vi "运维调试_总磷总氮.vi"() -> ()   [LabVIEW 2016, in "斯坦道总氮.lvlib"]
uses:
  <vilib>/Utility/miscctls.llb/LVPointTypeDef.ctl
  <vilib>/Plasmionique/MB Master/MB_Master/MB_Master.lvclass
  <vilib>/Utility/config.llb/NI_LVConfig.lvlib
  <vilib>/ptbypt/NI_PtbyPt.lvlib
panel:
  in  "关闭心跳包":bool
  out "权限等级":enum16{"一级权限", "二级权限", "三级权限", "超级权限"}(ring)
  out "试剂余量显示":sgl[][](graph)
  in  "仪器校准":bool
  in  "参数查询":bool
  out "简易步骤名称":string
  in  "温度曲线":bool
  in  "试剂余量":bool
  in  "灯值调整":bool
  in  "启动参数设置":bool
  out "固件版本号":string
  in  "定时设置":cluster{"启动":bool, "控制命令":T1, "测量参数":T2}(xcontrol)
  out "模块版本号":string
  out "注射器温度":sgl
  out "消解温度":sgl
  out "ADC":sgl
  out "F3":sgl format="%#.6f"
  out "F2":sgl format="%#.6f"
  out "F1":sgl format="%#.6f"
  out "F0":sgl format="%#.6f"
  out "运行状态":T3 {"数据时间:" format="%<%y/%m/%d %H:%M:%S>T"; "仪器时间:" format="%<%y/%m/%d %H:%M:%S>T"}
  in  "单选按钮":T4(radio)=enum."总氮"
  out "布尔":bool
  in  "流程固件":bool
  out "字符串 2":string
  in  "数组":string[](array[string])
  in  "返回":bool
  in  "参数设置":bool
  out "集成报警信息":string
  in  "停止":bool
  in  "手动启动":bool
  in  "调试":bool
  out "多列列表框":i32(listbox)
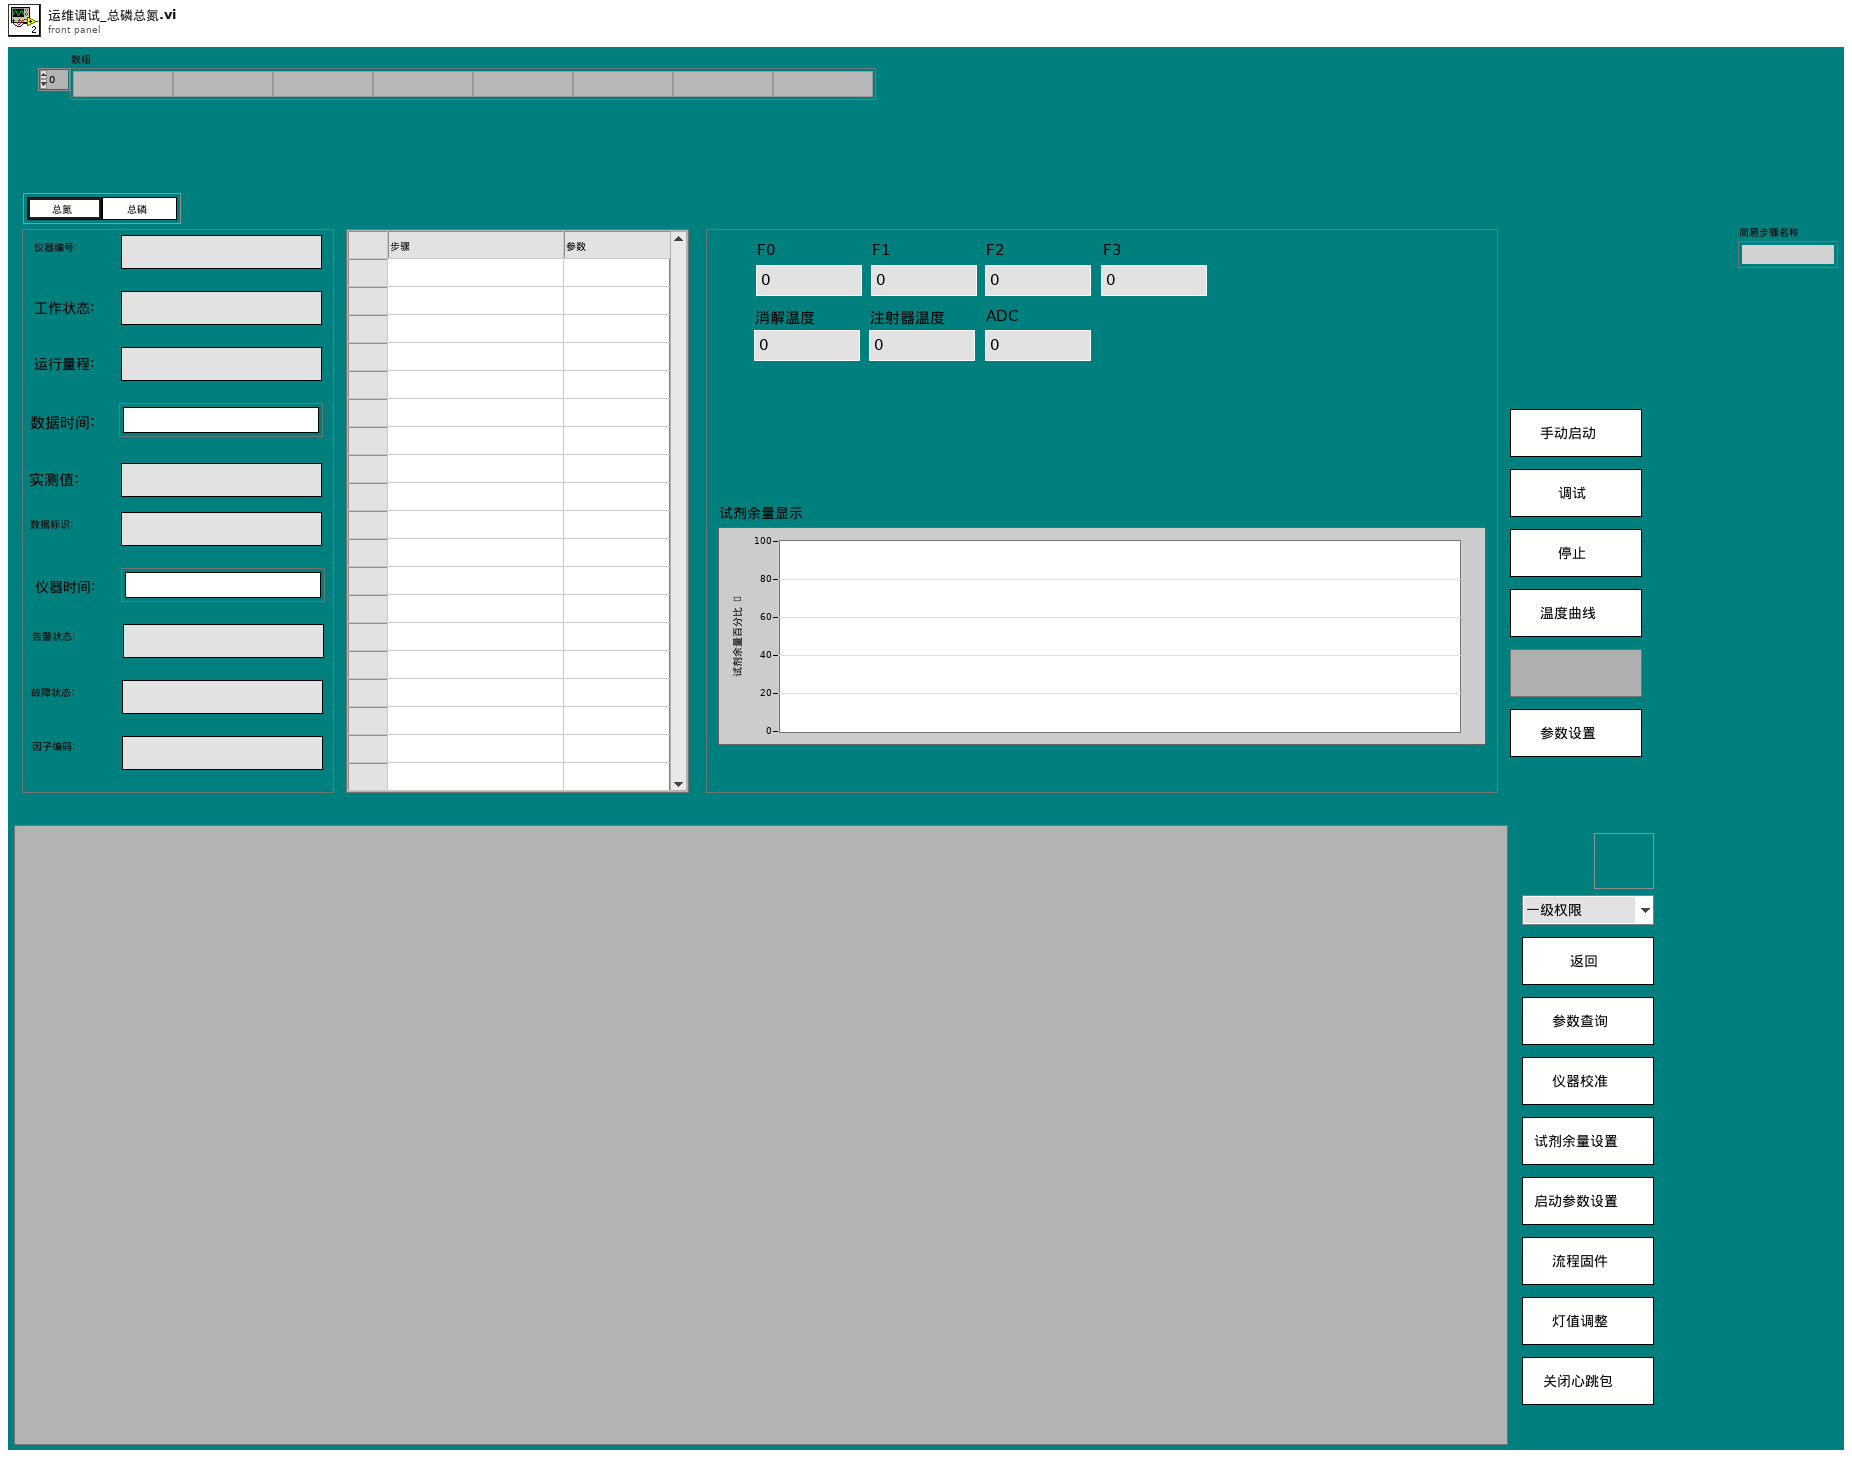
[diagram p1: front panel]
types:
  T1 = typedef "定时设置.xctl/国标控制命令.ctl" = enum16{"启动测量", "标样核查", "零点核查", "跨度核查", "空白测试", "平行样测试", "加标回收", "空白校准", "标样校准", "初始化（清洗）", "停止测试", "仪器重启", "校时", "模式设置", "测量间隔设置"}
  T2 = typedef "定时设置.xctl/测量参数.ctl" = u16
  T3 = cluster{"仪器编号:":string, "工作状态:":string, "运行量程: ":string, "数据时间:":timestamp, "实测值:":string, "数据标识: ":string, "仪器时间:":timestamp, "告警状态: ":string, "故障状态:  ":string, "因子编码:":string}
  T4 = enum32{"COD", "氨氮", "总氮", "总磷", "磷酸盐", "硝氮", "亚硝氮", "硅酸盐", "硫化物"}
  T5 = cluster{"时间源选择":enum16{"系统时间源", "仪器时间源"}, "外部时间源":timestamp}
  T6 = cluster{"系统时间":timestamp, "工作状态":u16, "测量模式":enum16{"待机", "连续模式", "周期模式", "定点模式", "受控模式", "手动模式"}, "告警代码":u16, "故障代码":u16, "日志代码":u16, "软件版本":u16, "F0":sgl, "F1":sgl, "F2":sgl, "F3":sgl, "T":sgl, "H":sgl, "id":u16, "flowid":u16, "量程":u16, "总磷控温温度1":sgl, "营养盐控温温度2":sgl, "ADC":sgl}
  T7 = enum32{"Bad", "Idle", "Run top level", "Running"}
  T8 = typedef "LVPointTypeDef.ctl" = cluster{"Horizontal":i16, "Vertical":i16}
  T9 = cluster{"因子编码":u32, "单位":u16, "标样参考值":sgl, "水样数据时间":timestamp, "水样实测值":sgl, "水样数据标识":string, "标样数据时间":timestamp, "标样实测值":sgl, "标样数据标识":string, "空白数据时间":timestamp, "空白实测值":sgl, "空白数据标识":string, "零点核查数据时间":timestamp, "零点核查实测值":sgl, "零点核查数据标识":string, "跨度核查数据时间":timestamp, "跨度核查实测值":sgl, "跨度核查数据标识":string, "加标回收数据时间":timestamp, "加标回收实测值":sgl, "加标回收数据标识":string, "平行样数据时间":timestamp, "平行样实测值":sgl, "平行样数据标识":string, "F0":sgl, "F1":sgl, "F2":sgl, "F3":sgl, "F4":sgl, "F5":sgl, "F6":sgl, "F7":sgl, "温度":sgl, "湿度":sgl, "X值":sgl, "fidrange":u16}[]
  T10 = cluster{"因子编码":u32, "单位":u16, "标样参考值":sgl, "水样数据时间":timestamp, "水样实测值":sgl, "水样数据标识":string, "标样数据时间":timestamp, "标样实测值":sgl, "标样数据标识":string, "空白数据时间":timestamp, "空白实测值":sgl, "空白数据标识":string, "零点核查数据时间":timestamp, "零点核查实测值":sgl, "零点核查数据标识":string, "跨度核查数据时间":timestamp, "跨度核查实测值":sgl, "跨度核查数据标识":string, "加标回收数据时间":timestamp, "加标回收实测值":sgl, "加标回收数据标识":string, "平行样数据时间":timestamp, "平行样实测值":sgl, "平行样数据标识":string, "F0":sgl, "F1":sgl, "F2":sgl, "F3":sgl, "F4":sgl, "F5":sgl, "F6":sgl, "F7":sgl, "温度":sgl, "湿度":sgl, "X值":sgl, "fidrange":u16}
  T11 = cluster{"时间标识":timestamp, "设备":string, "日志信息":string, "备注":string}
  T12 = cluster{"参数":string, "报警内容":string, "报警分析":string}
  T13 = cluster{"Major":u16, "Minor":u16, "Fix":u16, "Build":u16}
  T14 = typedef "NI_LVConfig.lvlib/Config Data RefNum.ctl" = refnum<k1>
  T15 = cluster{"时间标识":timestamp, "设备":string, "日志信息":string, "流程参数":string}
  T16 = typedef "LVRowAndColumnUnsignedTypeDef.ctl" = cluster{"Row":u32, "Column":u32}
  T17 = enum16{"空闲", "水样测试", "标样核查", "零点核查", "跨度核查", "空白测试", "平行样测试", "加标回收", "空白校准", "标样校准", "初始化（清洗）"}
  T18 = cluster{"站号":u16, "量程切换":enum32{"H", "L", "AUTO"}, "控制命令":enum16{"启动测量", "标样核查", "零点核查", "跨度核查", "空白测试", "平行样测试", "加标回收", "空白校准", "标样校准", "初始化（清洗）", "停止测试", "仪器重启", "校时", "模式设置", "测量间隔设置"}, "模式设置":enum16{"待机", "连续模式", "周期模式", "定点模式", "受控模式", "手动模式"}, "测量间隔":u16}
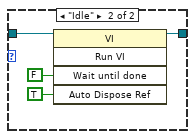
[diagram p4: hidden frame]
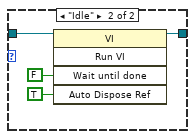
[diagram p5: hidden frame]
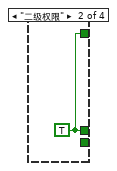
[diagram p13: hidden frame]
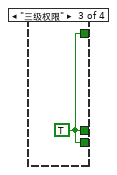
[diagram p14: hidden frame]
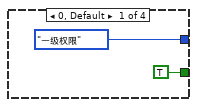
[diagram p15: hidden frame]
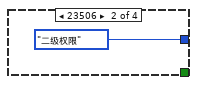
[diagram p16: hidden frame]
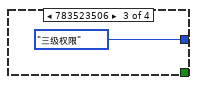
[diagram p17: hidden frame]
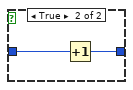
[diagram p19: hidden frame]
diagram:
  n1 = while {
    stop <- FALSE stop-if-true
    n2 = vi-ref "测量流程.vi"() -> (w49:refnum<vi>)
    n3 = global read "VAR总磷总氮全局变量.vi" "状态告警区"() -> (w46:T6)
    n4 = Wait (ms)(milliseconds to wait=u32 500 ("等待时间（毫秒）")) -> ()  [unwired: 1 out]
    n5 = Unbundle By Name("定时设置") -> ("启动"=w43:bool, "控制命令"=w42:T1)
    n6 = property class="VI"(reference=w49) -> ("Exec.State"=w48:T7, "Name"=w47:string)  [unwired: 1 in, 2 out]
    n7 = Unbundle By Name(w46) -> ("工作状态"=w45:u16, "系统时间"=w40:timestamp)
    n8 = case shown="真" w43 {
      tunnel: w47 -> [_ w56]
      tunnel: w42 -> [_ w55]
      tunnel: w48 -> [_ w54]
      frame False {
      }
      frame True {
        n9 = case shown="\"Idle\"" w54 {
          tunnel: w56 -> [_ w60]
          tunnel: w55 -> [_ w57]
          frame "Bad", Default {
          }
          frame "Idle" {
            n10 = Open VI Reference(type specifier VI Refnum (for type only)=refnum<vi> refnum, vi path=w60, options=128 ("选项")) -> (vi reference=w61:refnum<vi>, error out=w62:errorcluster)  [unwired: 3 in]
            n11 = call-by-ref "开始异步调用"(reference=w61, error in=w62, "控制命令"=w57) -> (reference out=w63:refnum<vi>, error out=w64:errorcluster)  [unwired: 11 in]
            n12 = Close Reference(reference=w63, error in (no error)=w64) -> ()  [unwired: 1 out]
          }
        }
      }
    }
    n13 = case shown="1, 默认" w45 {
      tunnel: [FALSE TRUE] -> w38
      frame 0 {
      }
      frame 1, Default {
      }
    }
    n14 = Bundle By Name(cluster=T5 {"时间源选择"=enum."仪器时间源", "外部时间源"=timestamp(0 s since 1904-01-01)} ("时间源"), "外部时间源"=w40) -> (w39:T5)
    n15 = property on="定时设置" class="定时设置 (严格)"("仪器状态"=w38, "时间源"=w39) -> ()  [unwired: 2 in, 2 out]
  }
  n16 = control-ref of="本VI"() -> (w20:refnum<vi>)
  n17 = call "配置文件路径.vi"() -> ("appended path"=w31:path)  [unwired: 11 in]
  n18 = call "时间延迟"() -> ("error out"=w37:errorcluster)  [unwired: 11 in]
  n19 = flat-sequence {
    frame #0 {
      n20 = property on="窗格" class="Pane"("Origin"=T8 {"Horizontal"=0, "Vertical"=0} ("原点")) -> ()  [unwired: 2 in, 2 out]
    }
  }
  n21 = while {
    shift-right: [w68] -> _
    shift-left: _ -> [w67]
    stop <- FALSE stop-if-true
    n22 = global write "VAR总磷总氮全局变量.vi" "最近一次工作状态"(w67) -> ()
    n23 = global read "VAR总磷总氮全局变量.vi" "状态告警区"() -> (w90:T6)
    n24 = global read "VAR总磷总氮全局变量.vi" "通讯状态"() -> (w101:bool)
    n25 = Wait (ms)(milliseconds to wait=u32 1000 ("等待时间（毫秒）")) -> ()  [unwired: 1 out]
    n26 = case shown="\"COD\", 默认" "单选按钮" {
      tunnel: [22 3 2 1 4 5 6 7 8] -> w69
      frame "COD", Default {
      }
      frame "氨氮" {
      }
      frame "总氮" {
      }
      frame "总磷" {
      }
      frame "磷酸盐" {
      }
      frame "硝氮" {
      }
      frame "亚硝氮" {
      }
      frame "硅酸盐" {
      }
      frame "硫化物" {
      }
    }
    n27 = Unbundle By Name(w90) -> ("id"=w89:u16, "工作状态"=w84:u16)
    n28 = case shown="真" w101 {
      tunnel: ["通讯异常" ("集成报警信息") w195] -> w100
      frame False {
      }
      frame True {
        n29 = global read "VAR总磷总氮全局变量.vi" "状态告警区"() -> (w201:T6)
        n30 = Unbundle By Name(w201) -> ("工作状态"=w200:u16)
        n31 = feedback #1(0) -> (w198:i32)
        n32 = case shown="默认" w200 {
          tunnel: w198 -> [_ w203]
          tunnel: [_ w202] -> w196
          frame 0 {
          }
          frame Default {
            n33 = Increment(x=w203) -> (x+1=w202:i32)
          }
        }
        n34 = feedback-in #1(w196) -> ()
        n35 = global read "VAR总磷总氮全局变量.vi" "测量状态"() -> (w194:string)
        n36 = Format Into String(format string="工作计时: %d 秒" ("格式字符串"), initial string=w194, w196) -> (resulting string=w195:string)  [unwired: 1 in, 1 out]
      }
    }
    "集成报警信息" <- w100
    n37 = global read "VAR总磷总氮全局变量.vi" "测量数据区数组"() -> (w73:T9)
    n38 = case shown="1, 默认" w84 {
      tunnel: w89 -> [_ w146]
      frame 0 {
      }
      frame 1, Default {
        n39 = case shown="8" w146 {
          frame 0, Default {
          }
          frame 1 {
            n40 = local write "单选按钮"(T4."总磷" ("单选按钮")) -> ()
          }
          frame 2 {
            n41 = local write "单选按钮"(T4."总氮" ("单选按钮")) -> ()
          }
          frame 22 {
            n42 = local write "单选按钮"(T4."COD" ("单选按钮")) -> ()
          }
          frame 3 {
            n43 = local write "单选按钮"(T4."氨氮" ("单选按钮")) -> ()
          }
          frame 4 {
            n44 = local write "单选按钮"(T4."磷酸盐" ("单选按钮")) -> ()
          }
          frame 5 {
            n45 = local write "单选按钮"(T4."硝氮" ("单选按钮")) -> ()
          }
          frame 6 {
            n46 = local write "单选按钮"(T4."亚硝氮" ("单选按钮")) -> ()
          }
          frame 7 {
            n47 = local write "单选按钮"(T4."硅酸盐" ("单选按钮")) -> ()
          }
          frame 8 {
            n48 = local write "单选按钮"(T4."硫化物" ("单选按钮")) -> ()
          }
        }
      }
    }
    n49 = call "id参数转换.vi"("id"=w69) -> ("数组资源索引"=w70:i32)  [unwired: 9 in, 1 out]
    n50 = global read "VAR总磷总氮全局变量.vi" "状态告警区"() -> (w99:T6)
    n51 = Index Array(array=w73, index=w70) -> (element=w72:T10)
    n52 = Unbundle By Name(w99) -> ("系统时间"=w95:timestamp, "工作状态"=w94:u16, "告警代码"=w88:u16, "故障代码"=w86:u16, "量程"=w93:u16)
    n53 = case shown="5, 8" w67 {
      tunnel: [w115 w121 w125 w129 w133 w137 w141 w145] -> w83
      tunnel: [w113 w120 w124 w128 w131 w136 w140 w144] -> w78
      tunnel: [w116 w119 w123 w127 w130 w135 w139 w143] -> w76
      tunnel: w72 -> [_ w118 w122 w126 w132 w134 w138 w142]
      frame 0, Default {
        n54 = local read "运行状态"() -> (w117:T3)
        n55 = Unbundle By Name(w117) -> ("数据时间:"=w115:timestamp, "实测值:"=w114:string, "数据标识:"=w116:string)
        n56 = Fract/Exp String To Number(string=w114) -> (number=w113:dbl)  [unwired: 3 in, 1 out]
      }
      frame 1 {
        n57 = Unbundle By Name(w118) -> ("水样数据时间"=w121:timestamp, "水样实测值"=w120:sgl, "水样数据标识"=w119:string)
      }
      frame 2, 9 {
        n58 = Unbundle By Name(w122) -> ("标样数据时间"=w125:timestamp, "标样实测值"=w124:sgl, "标样数据标识"=w123:string)
      }
      frame 3 {
        n59 = Unbundle By Name(w126) -> ("零点核查数据时间"=w129:timestamp, "零点核查实测值"=w128:sgl, "零点核查数据标识"=w127:string)
      }
      frame 4 {
        n60 = Unbundle By Name(w132) -> ("跨度核查数据时间"=w133:timestamp, "跨度核查实测值"=w131:sgl, "跨度核查数据标识"=w130:string)
      }
      frame 7 {
        n61 = Unbundle By Name(w134) -> ("加标回收数据时间"=w137:timestamp, "加标回收实测值"=w136:sgl, "加标回收数据标识"=w135:string)
      }
      frame 5, 8 {
        n62 = Unbundle By Name(w138) -> ("空白数据时间"=w141:timestamp, "空白实测值"=w140:sgl, "空白数据标识"=w139:string)
      }
      frame 6 {
        n63 = Unbundle By Name(w142) -> ("平行样数据时间"=w145:timestamp, "平行样实测值"=w144:sgl, "平行样数据标识"=w143:string)
      }
    }
    n64 = Unbundle By Name(w72) -> ("因子编码"=w74:u32)
    n65 = case shown="255" w94 {
      selector: w94 -> [w160 _ w166 w168 w170 w172 w174 w176 w178 w180 w182 w184 w186 w188]
      tunnel: [w161 "空闲" ("工作状态") "水样测量" ("工作状态") "标样核查" ("工作状态") "零点核查" ("工作状态") "跨度核查" ("工作状态") "空白测试" ("工作状态") "平行样测试" ("工作状态") "加标回收" ("工作状态") "空白校准" ("工作状态") "标样校准" ("工作状态") "初始化" ("工作状态") "单步调试" ("工作状态") w190] -> w66
      tunnel: [w159 w164 w166 w168 w170 w172 w174 w176 w178 w180 w182 w184 w186 w188] -> w68
      tunnel: w67 -> [w159 w164 _ _ _ _ _ _ _ _ _ _ _ _]
      frame Default {
        n66 = Format Into String(format string="%d" ("格式字符串"), initial string="未知" ("工作状态"), w160) -> (resulting string=w161:string)  [unwired: 1 in, 1 out]
      }
      frame 0 {
      }
      frame 1 {
      }
      frame 2 {
      }
      frame 3 {
      }
      frame 4 {
      }
      frame 5 {
      }
      frame 6 {
      }
      frame 7 {
      }
      frame 8 {
      }
      frame 9 {
      }
      frame 10 {
      }
      frame 254 {
      }
      frame 255 {
        n67 = local read "简易步骤名称"() -> (w191:string)
        n68 = Format Into String(format string="-%d (%s)" ("格式字符串"), initial string="简易流程" ("工作状态"), w188, w191) -> (resulting string=w190:string)  [unwired: 1 in, 1 out]
      }
    }
    n69 = case shown="1" w93 {
      tunnel: ["" ("字符串") "低量程 " ("字符串") "高量程 " ("字符串")] -> w92
      frame Default {
      }
      frame 0 {
      }
      frame 1 {
      }
    }
    n70 = Number To Fractional String(number=w78, precision (6)=i16 4 ("精度(6)")) -> (F-format string=w80:string)  [unwired: 2 in]
    n71 = Concatenate Strings(w80, " " ("字符串"), "mg/L" ("字符串")) -> (w77:string)
    n72 = global read "VAR总磷总氮全局变量.vi" "序列号"() -> (w96:string)
    n73 = Format Into String(format string="w%05d" ("格式字符串"), w74) -> (resulting string=w91:string)  [unwired: 2 in, 1 out]
    n74 = call "告警码字段定义.vi"("告警代码"=w88) -> ("字符串"=w87:string)  [unwired: 8 in, 2 out]
    n75 = call "故障码字段定义.vi"("故障代码"=w86) -> ("字符串"=w85:string)  [unwired: 10 in]
    n76 = global write "VAR总磷总氮全局变量.vi" "工作状态:"(w66) -> ()
    n77 = Bundle By Name(cluster=T3 {"仪器编号:"="", "工作状态:"="", "运行量程: "="", "数据时间:"=timestamp(0 s since 1904-01-01), "实测值:"="", "数据标识: "="", "仪器时间:"=timestamp(0 s since 1904-01-01), "告警状态: "="", "故障状态:  "="", "因子编码:"=""} ("运行状态"), "仪器编号:"=w96, "仪器时间:"=w95, "工作状态:"=w66, "告警状态:"=w87, "故障状态:"=w85, "运行量程:"=w92, "数据时间:"=w83, "实测值:"=w77, "数据标识:"=w76, "因子编码:"=w91) -> (→"运行状态":T3)
  }
  n78 = call "Create balloon 队列.vi"() -> ("队列输出"=w34:refnum<queue>)  [unwired: 11 in]
  n79 = while {
    shift-right: [w207] -> _
    shift-left: _ -> [w206]
    stop <- FALSE stop-if-true
    n80 = global read "VAR总磷总氮全局变量.vi" "状态告警区"() -> (w209:T6)
    n81 = Wait (ms)(milliseconds to wait=u32 1000 ("等待时间（毫秒）")) -> ()  [unwired: 1 out]
    n82 = Unbundle By Name(w209) -> ("工作状态"=w208:u16, "总磷控温温度1"=w205:sgl, "营养盐控温温度2"=w204:sgl)
    n83 = case shown="默认" w208 {
      tunnel: [TRUE _] -> w207
      tunnel: w206 -> [w218 _]
      tunnel: w205 -> [w216 _]
      tunnel: w204 -> [w214 _]
      frame Default {
        n84 = case shown="真" w218 {
          tunnel: [_ w221] -> w217
          tunnel: [_ w220] -> w215
          frame False {
          }
          frame True {
            n85 = global read "VAR总磷总氮全局变量.vi" "波形图-消解温度"() -> (w221:dbl[])
            n86 = global read "VAR总磷总氮全局变量.vi" "波形图-注射器温度"() -> (w220:dbl[])
          }
        }
        n87 = Insert Into Array(array=w217, new element=w216) -> (w213:dbl[])  [unwired: 1 in]
        n88 = Insert Into Array(array=w215, new element=w214) -> (w212:dbl[])  [unwired: 1 in]
        n89 = global write "VAR总磷总氮全局变量.vi" "波形图-消解温度"(w213) -> ()
        n90 = global write "VAR总磷总氮全局变量.vi" "波形图-注射器温度"(w212) -> ()
      }
      frame 0, 254, 255 {
      }
    }
  }
  n91 = while {
    stop <- FALSE stop-if-true
    n92 = control-ref of="试剂余量显示"() -> (w223:refnum<vi>)
    n93 = Wait (ms)(milliseconds to wait=u32 10000 ("等待时间（毫秒）")) -> ()  [unwired: 1 out]
    n94 = call "试剂余量展示.vi"("波形图 2"=w223) -> ("波形图"=→"试剂余量显示":sgl[][])  [unwired: 10 in]
  }
  n95 = call "试剂余量后台任务.vi"() -> ()  [unwired: 12 in]
  n96 = while {
    shift-right: [w238] -> _
    shift-left: u32 0 ("y") -> [w240]
    stop <- FALSE stop-if-true
    # "密码权限"
    n97 = local read "布尔"() -> (w241:bool)
    n98 = global read "VAR总磷总氮全局变量.vi" "权限密码"() -> (w233:u32)
    n99 = global read "VAR总磷总氮全局变量.vi" "权限等级"() -> (w230:enum16{"一级权限", "二级权限", "三级权限", "超级权限"})
    n100 = global read "VAR总磷总氮全局变量.vi" "权限等级"() -> (→"权限等级":enum16{"一级权限", "二级权限", "三级权限", "超级权限"})
    n101 = Wait (ms)(milliseconds to wait=u32 1000 ("等待时间（毫秒）")) -> ()  [unwired: 1 out]
    n102 = case shown="假" w241 {
      tunnel: w240 -> [_ w254]
      tunnel: [_ w253] -> w238
      frame False {
      }
      frame True {
        n103 = Increment(x=w254) -> (x+1=w253:u32)
      }
    }
    n104 = case shown="783523103" w233 {
      tunnel: [enum16{"一级权限", "二级权限", "三级权限", "超级权限"}."一级权限" ("权限等级") enum16{"一级权限", "二级权限", "三级权限", "超级权限"}."二级权限" ("权限等级") enum16{"一级权限", "二级权限", "三级权限", "超级权限"}."三级权限" ("权限等级") enum16{"一级权限", "二级权限", "三级权限", "超级权限"}."超级权限" ("权限等级")] -> w234
      tunnel: [TRUE _ _ _] -> w232
      frame 0, Default {
      }
      frame 23506 {
      }
      frame 783523506 {
      }
      frame 783523103 {
      }
    }
    n105 = case shown="\"超级权限\"" w230 {
      tunnel: [_ w243 w244 w246] -> w227
      tunnel: [_ _ w244 w246] -> w229
      tunnel: [_ w243 w244 w246] -> w228
      tunnel: [_ _ _ TRUE] -> w226
      frame "一级权限", Default {
      }
      frame "二级权限" {
        w243 = TRUE
      }
      frame "三级权限" {
        w244 = TRUE
      }
      frame "超级权限" {
        w246 = TRUE
      }
    }
    n106 = Greater Or Equal?(x=w238, y=u32 3600) -> (x >= y?=w236:bool)
    n107 = property on="关闭心跳包" class="Bool (严格)"("Visible"=w226) -> ()  [unwired: 2 in, 2 out]
    n108 = case shown="真" w236 {
      frame False {
      }
      frame True {
        n109 = global write "VAR总磷总氮全局变量.vi" "权限密码"(u32 0 ("权限密码")) -> ()
      }
    }
    n110 = property on="流程固件" class="Bool"("Visible"=w228) -> ()  [unwired: 2 in, 2 out]
    n111 = property on="试剂余量" class="Bool"("Visible"=w227) -> ()  [unwired: 2 in, 2 out]
    n112 = property on="灯值调整" class="Bool"("Visible"=w227) -> ()  [unwired: 2 in, 2 out]
    n113 = property on="启动参数设置" class="Bool"("Visible"=w229) -> ()  [unwired: 2 in, 2 out]
    n114 = global write "VAR总磷总氮全局变量.vi" "权限等级"(w234) -> ()
    n115 = Not(x=w232) -> (.not. x?=→"布尔":bool)
  }
  n116 = while {
    tunnel: w34 -> [w261]
    shift-right: [w257] -> _
    shift-left: _ -> [w258]
    stop <- FALSE stop-if-true
    n117 = global read "VAR总磷总氮全局变量.vi" "状态告警区"() -> (w255:T6)
    n118 = Wait (ms)(milliseconds to wait=u32 100) -> ()  [unwired: 1 out]
    n119 = Unbundle By Name(w255) -> ("工作状态"=w256:u16, "id"=w263:u16, "日志代码"=w262:u16, "故障代码"=w260:u16, "告警代码"=w259:u16)
    n120 = case shown="1, 默认" w256 {
      tunnel: w263 -> [_ w278]
      tunnel: w262 -> [_ w277]
      tunnel: w261 -> [_ w274]
      tunnel: w260 -> [_ w273]
      tunnel: w259 -> [_ w272]
      tunnel: w258 -> [w266 w271]
      tunnel: [w266 w270] -> w257
      frame 0 {
      }
      frame 1, Default {
        n121 = call "id参数转换.vi"("id"=w278) -> ("table输出"=w275:string)  [unwired: 9 in, 1 out]
        n122 = Add(x=w273, y=w272) -> (x+y=w270:u16)
        n123 = Not Equal?(x=w270, y=w271) -> (x != y?=w268:bool)
        n124 = Not Equal To 0?(x=w270) -> (x != 0?=w269:bool)
        n125 = call "故障告警分析.vi"("告警代码"=w272, "故障代码"=w273, "运行步序"=w277, "参数"=w275) -> ("报警内容"=w276:T12)  [unwired: 6 in, 1 out]
        n126 = And(x=w269, y=w268) -> (x .and. y?=w267:bool)
        n127 = case shown="真" w267 {
          tunnel: w276 -> [_ w287]
          tunnel: w274 -> [_ w286]
          frame False {
          }
          frame True {
            n128 = Unbundle By Name(w287) -> ("参数"=w282:string, "报警内容"=w281:string, "报警分析"=w280:string)
            n129 = Get Date/Time In Seconds() -> (seconds since 1Jan1904=w285:timestamp)
            n130 = Bundle("报警内容"=w281, "报警分析"=w280) -> (w279:cluster{"报警内容":string, "报警分析":string})  [unwired: 1 in]
            n131 = Bundle By Name(cluster=T11 {"时间标识"=timestamp(0 s since 1904-01-01), "设备"="", "日志信息"="", "备注"=""} ("data in"), "时间标识"=w285, "设备"=w282, "日志信息"=w281, "备注"=w280) -> (w284:T11)
            n132 = call "balloon入队列.vi"("报警内容"=w279, "队列"=w286) -> ()  [unwired: 9 in, 1 out]
            n133 = call "总磷总氮报警信息.vi"("data in"=w284) -> ()  [unwired: 10 in, 1 out]
          }
        }
      }
    }
  }
  n134 = Read from Text File(file (use dialog)=w31) -> (text=w32:string)  [unwired: 3 in, 3 out]
  n135 = flat-sequence {
    tunnel: [w289] -> w26
    tunnel: [w288] -> w24
    tunnel: w26 -> [w300]
    tunnel: [w300] -> w25
    tunnel: w24 -> [_]
    tunnel: w25 -> [w330]
    tunnel: [w330] -> w27
    tunnel: w27 -> [w333]
    tunnel: [w403] -> w28
    tunnel: [errorcluster {"status"=FALSE, "code"=0, "source"=""} ("错误输入（无错误）")] -> w3
    tunnel: [errorcluster {"status"=FALSE, "code"=0, "source"=""} ("错误输入（无错误）")] -> w2
    frame #0 {
      n136 = call "配置读取.vi"() -> ("error out"=w288:errorcluster)  [unwired: 11 in]
      n137 = control-ref of="本VI"() -> (w299:refnum<vi>)
      n138 = property class="VI"(reference=w299) -> ("Library.Version"=w298:T13)  [unwired: 1 in, 2 out]
      n139 = Unbundle By Name(w298) -> ("Major"=w296:u16, "Minor"=w295:u16, "Fix"=w294:u16, "Build"=w293:u16)
      n140 = control-ref of="本VI"() -> (w290:refnum<vi>)
      n141 = property class="VI"(reference=w290) -> ("Library"=w291:refnum<vi>)  [unwired: 1 in, 2 out]
      n142 = Format Into String(format string="模块版本号：%d.%d.%d.%d" ("格式字符串"), w296, w295, w294, w293) -> (resulting string=→"模块版本号":string)  [unwired: 2 in, 1 out]
      n143 = property class="Library"(reference=w291) -> ("LocalName"=w289:string)  [unwired: 1 in, 2 out]
      n144 = property on="定时设置" class="定时设置 (严格)"("引用参数"=w289) -> ()  [unwired: 2 in, 2 out]
    }
    frame #1 {
      n145 = global read "总磷总氮断电保存全局变量.vi" "IP"() -> (w304:string)
      n146 = global read "总磷总氮断电保存全局变量.vi" "VISA Resource"() -> (w301:refnum<visa-resource-name>)
      n147 = Empty String/Path?(string/path=w304) -> (empty?=w303:bool)
      n148 = case shown="真" w303 {
        tunnel: w300 -> [_ w315]
        frame False {
        }
        frame True {
          n149 = case shown="\"斯坦道CODcr.lvlib\"" w315 {
            tunnel: [w316 "192.168.1.203" ("IP") "192.168.1.202" ("IP") "192.168.1.202" ("IP") "192.168.1.203" ("IP") "192.168.1.204" ("IP") "192.168.1.205" ("IP")] -> w314
            frame Default {
              n150 = global read "总磷总氮断电保存全局变量.vi" "IP"() -> (w316:string)
            }
            frame "斯坦道总磷总氮.lvlib" {
            }
            frame "斯坦道氨氮.lvlib" {
            }
            frame "斯坦道氨氮总磷.lvlib" {
            }
            frame "斯坦道总磷.lvlib" {
            }
            frame "斯坦道总氮.lvlib" {
            }
            frame "斯坦道CODcr.lvlib" {
            }
          }
          n151 = global write "总磷总氮断电保存全局变量.vi" "IP"(w314) -> ()
        }
      }
      n152 = Empty String/Path?(string/path=w301) -> (empty?=w302:bool)
      n153 = case shown="真" w302 {
        tunnel: w300 -> [_ w306]
        frame False {
        }
        frame True {
          n154 = case shown="\"斯坦道总氮.lvlib\"" w306 {
            tunnel: [w307 "COM5" ("IP") "COM7" ("IP") "COM7" ("IP") "COM5" ("IP") "COM10" ("IP") "COM9" ("IP")] -> w305
            frame Default {
              n155 = global read "总磷总氮断电保存全局变量.vi" "VISA Resource"() -> (w307:refnum<visa-resource-name>)
            }
            frame "斯坦道总磷总氮.lvlib" {
            }
            frame "斯坦道氨氮.lvlib" {
            }
            frame "斯坦道氨氮总磷.lvlib" {
            }
            frame "斯坦道总磷.lvlib" {
            }
            frame "斯坦道总氮.lvlib" {
            }
            frame "斯坦道CODcr.lvlib" {
            }
          }
          n156 = global write "总磷总氮断电保存全局变量.vi" "VISA Resource"(w305) -> ()
        }
      }
    }
    frame #2 {
      n157 = global read "总磷总氮断电保存全局变量.vi" "MB通信方式选择"() -> (w326:enum16{"串口", "TCP"})
      n158 = global read "总磷总氮断电保存全局变量.vi" "VISA Resource"() -> (w325:refnum<visa-resource-name>)
      n159 = global read "总磷总氮断电保存全局变量.vi" "PORT"() -> (w328:string)
      n160 = Decimal String To Number(string=w328) -> (number=w327:i32)  [unwired: 2 in, 1 out]
      n161 = global read "总磷总氮断电保存全局变量.vi" "IP"() -> (w329:string)
      n162 = call "获取启动参数.vi"("MB通信方式选择"=w326, "Port (502)"=w327, "IP Address"=w329, "VISA Resource"=w325) -> ("error out"=w324:errorcluster, "数组"=w323:cluster{"String":string, "Value":u16}[])  [unwired: 6 in]
      n163 = case shown="无错误" w324 {
        tunnel: w323 -> [w331 _]
        frame No Error {
          n164 = flat-sequence {
            tunnel: w331 -> [w332]
            frame #0 {
              n165 = global write "总磷总氮断电保存全局变量.vi" "启动队列名称"(w332) -> ()
            }
            frame #1 {
              n166 = call "配置写入.vi"() -> ()  [unwired: 11 in, 1 out]
            }
          }
        }
        frame Error {
        }
      }
    }
    frame #3 {
      n167 = global read "总磷总氮断电保存全局变量.vi" "启动队列名称"() -> (w335:cluster{"String":string, "Value":u16}[])
      n168 = Empty Array?(array=w335) -> (empty?=w334:bool)
      n169 = case shown="真" w334 {
        tunnel: w333 -> [_ w336]
        frame False {
        }
        frame True {
          n170 = case shown="\"斯坦道总氮.lvlib\"" w336 {
            frame Default {
            }
            frame "斯坦道总磷总氮.lvlib" {
              n171 = global write "总磷总氮断电保存全局变量.vi" "启动队列名称"(cluster{"String":string, "Value":u16}[] [{"String"="总氮", "Value"=2}, {"String"="总磷", "Value"=1}] ("启动队列名称")) -> ()
            }
            frame "斯坦道氨氮.lvlib" {
              n172 = global write "总磷总氮断电保存全局变量.vi" "启动队列名称"(cluster{"String":string, "Value":u16}[] [{"String"="氨氮", "Value"=3}] ("启动队列名称")) -> ()
            }
            frame "斯坦道氨氮总磷.lvlib" {
              n173 = global write "总磷总氮断电保存全局变量.vi" "启动队列名称"(cluster{"String":string, "Value":u16}[] [{"String"="氨氮", "Value"=3}, {"String"="总磷", "Value"=1}] ("启动队列名称")) -> ()
            }
            frame "斯坦道总磷.lvlib" {
              n174 = global write "总磷总氮断电保存全局变量.vi" "启动队列名称"(cluster{"String":string, "Value":u16}[] [{"String"="总磷", "Value"=1}] ("启动队列名称")) -> ()
            }
            frame "斯坦道总氮.lvlib" {
              n175 = global write "总磷总氮断电保存全局变量.vi" "启动队列名称"(cluster{"String":string, "Value":u16}[] [{"String"="总氮", "Value"=2}] ("启动队列名称")) -> ()
            }
            frame "斯坦道CODcr.lvlib" {
              n176 = global write "总磷总氮断电保存全局变量.vi" "启动队列名称"(cluster{"String":string, "Value":u16}[] [{"String"="CODcr", "Value"=22}] ("启动队列名称")) -> ()
            }
          }
        }
      }
    }
    frame #4 {
      # "初始化"
      n177 = global read "总磷总氮断电保存全局变量.vi" "简易流程路径"() -> (w344:path)
      n178 = global read "总磷总氮断电保存全局变量.vi" "流程路径"() -> (w347:path)
      n179 = global read "总磷总氮断电保存全局变量.vi" "启动队列名称"() -> (w357:cluster{"String":string, "Value":u16}[])
      n180 = global read "总磷总氮断电保存全局变量.vi" "启动队列名称"() -> (w355:cluster{"String":string, "Value":u16}[])
      n181 = call <vilib>:"Check if File or Folder Exists.vi"("path"=w347) -> ("file or folder exists?"=w352:bool)  [unwired: 8 in, 2 out]
      n182 = call <vilib>:"Check if File or Folder Exists.vi"("path"=w344) -> ("file or folder exists?"=w351:bool)  [unwired: 8 in, 2 out]
      n183 = for {
        tunnel: w357 -> [w374] mode=indexing
        tunnel: [w373] -> w356 mode=indexing
        n184 = Unbundle By Name(w374) -> ("String"=w373:string)
      }
      n185 = Not(x=w351) -> (.not. x?=w346:bool)
      n186 = Not(x=w352) -> (.not. x?=w350:bool)
      n187 = Empty String/Path?(string/path=w344) -> (empty?=w343:bool)
      n188 = for {
        tunnel: w355 -> [w372] mode=indexing
        shift-right: [w371] -> w354
        shift-left: "" -> [w369]
        n189 = Unbundle By Name(w372) -> ("String"=w370:string)
        n190 = Concatenate Strings(w369, w370) -> (w371:string)
      }
      n191 = Empty String/Path?(string/path=w347) -> (empty?=w348:bool)
      n192 = Or(x=w343, y=w346) -> (x .or. y?=w345:bool)
      n193 = Or(x=w348, y=w350) -> (x .or. y?=w349:bool)
      n194 = property on="单选按钮" class="RadioBtnsControl (严格)"() -> ("Controls[]"=w358:refnum<vi>[])  [unwired: 2 in, 2 out]
      n195 = for {
        tunnel: w358 -> [w382] mode=indexing
        tunnel: w356 -> [w381]
        n196 = property class="Ctl"(reference=w382) -> (reference out=w380:refnum<vi>, "Label.Text"=w376:string)  [unwired: 1 in, 1 out]
        n197 = case shown="\"COD\"" w376 {
          selector: w376 -> [w383 _]
          tunnel: [w383 "CODcr"] -> w375
          frame Default {
          }
          frame "COD" {
          }
        }
        n198 = Search 1D Array(1D array=w381, element=w375) -> (index of element=w379:i32)  [unwired: 1 in]
        n199 = Not Equal?(x=w379, y=-1) -> (x != y?=w377:bool)
        n200 = property class="Ctl"(reference=w380, "Visible"=w377) -> ()  [unwired: 1 in, 2 out]
      }
      n201 = case shown="真" w345 {
        frame False {
        }
        frame True {
          n202 = global read "总磷总氮断电保存全局变量.vi" "启动队列名称"() -> (w360:cluster{"String":string, "Value":u16}[])
          n203 = for {
            tunnel: w360 -> [w363] mode=indexing
            tunnel: [w362] -> w359 mode=indexing
            n204 = Unbundle By Name(w363) -> ("String"=w362:string)
          }
          n205 = call "获取默认流程路径.vi"("参数"=w359) -> ("路径"=w361:path)  [unwired: 10 in]
          n206 = global write "总磷总氮断电保存全局变量.vi" "简易流程路径"(w361) -> ()
        }
      }
      n207 = case shown="真" w349 {
        frame False {
        }
        frame True {
          n208 = global read "总磷总氮断电保存全局变量.vi" "启动队列名称"() -> (w365:cluster{"String":string, "Value":u16}[])
          n209 = for {
            tunnel: w365 -> [w368] mode=indexing
            tunnel: [w367] -> w364 mode=indexing
            n210 = Unbundle By Name(w368) -> ("String"=w367:string)
          }
          n211 = call "获取默认流程路径.vi"("参数"=w364) -> ("路径"=w366:path)  [unwired: 10 in]
          n212 = global write "总磷总氮断电保存全局变量.vi" "流程路径"(w366) -> ()
        }
      }
      n213 = global write "VAR总磷总氮全局变量.vi" "模块名称"(w354) -> ()
    }
    frame #5 {
      n214 = vi-ref "总磷总氮通讯.vi"() -> (w385:refnum<vi>)
      n215 = vi-ref "总磷总氮测量数据储存.vi"() -> (w393:refnum<vi>)
      n216 = property class="VI"(reference=w385) -> ("Name"=w386:string)  [unwired: 1 in, 2 out]
      n217 = property class="VI"(reference=w393) -> ("Name"=w400:string)  [unwired: 1 in, 2 out]
      n218 = Open VI Reference(type specifier VI Refnum (for type only)=refnum<vi> refnum, vi path=w386, options=128 ("选项")) -> (vi reference=w388:refnum<vi>, error out=w390:errorcluster)  [unwired: 3 in]
      n219 = call-by-ref "开始异步调用"(reference=w388, error in=w390) -> (reference out=w392:refnum<vi>, error out=w391:errorcluster)  [unwired: 12 in]
      n220 = Open VI Reference(type specifier VI Refnum (for type only)=refnum<vi> refnum, vi path=w400, options=128 ("选项")) -> (vi reference=w398:refnum<vi>, error out=w396:errorcluster)  [unwired: 3 in]
      n221 = Close Reference(reference=w392, error in (no error)=w391) -> ()  [unwired: 1 out]
      n222 = call-by-ref "开始异步调用"(reference=w398, error in=w396) -> (reference out=w394:refnum<vi>, error out=w395:errorcluster)  [unwired: 12 in]
      n223 = Close Reference(reference=w394, error in (no error)=w395) -> ()  [unwired: 1 out]
    }
    frame #6 {
      n224 = call "设置模块队列名.vi"() -> ("Msg"=w403:string)  [unwired: 5 in]
    }
  }
  n225 = property class="VI"(reference=w20) -> ("Library"=w21:refnum<vi>)  [unwired: 1 in, 2 out]
  n226 = while {
    shift-right: [w407] -> _
    shift-left: w32 -> [w409]
    tunnel: w31 -> [w406]
    tunnel: [w404] -> _
    stop <- FALSE stop-if-true
    n227 = Read from Text File(file (use dialog)=w406) -> (text=w407:string, error out=w404:errorcluster)  [unwired: 3 in, 2 out]
    n228 = Not Equal?(x=w409, y=w407) -> (x != y?=w408:bool)
    n229 = Wait (ms)(milliseconds to wait=u32 1000 ("等待时间（毫秒）")) -> ()  [unwired: 1 out]
    n230 = case shown="真" w408 {
      tunnel: w406 -> [_ w412]
      tunnel: [_ w411] -> _
      frame False {
      }
      frame True {
        n231 = vi-ref "总磷总氮断电保存全局变量.vi"() -> (w416:refnum<vi>)
        n232 = call <vilib>:"Open Config Data.vi"("configuration file path"=w412) -> ("error out"=w414:errorcluster, "refnum"=w417:T14)  [unwired: 8 in, 1 out]
        n233 = call <userlib>:"Read Panel from INI__ogtk.vi"("error in (no error)"=w414, "VI ref"=w416, "refnum"=w417) -> ("error out"=w413:errorcluster, "refnum out"=w415:T14)  [unwired: 7 in]
        n234 = call <vilib>:"Close Config Data.vi"("error in (no error)"=w413, "refnum"=w415) -> ("error out"=w411:errorcluster)  [unwired: 8 in, 1 out]
      }
    }
  }
  n235 = property class="Library"(reference=w21) -> ("LocalName"=w18:string)  [unwired: 1 in, 2 out]
  n236 = while {
    tunnel: w37 -> [_]
    stop <- FALSE stop-if-true
    n237 = global read "VAR总磷总氮全局变量.vi" "状态告警区"() -> (w446:T6)
    n238 = global read "VAR总磷总氮全局变量.vi" "状态告警区"() -> (w445:T6)
    n239 = global read "VAR总磷总氮全局变量.vi" "状态告警区"() -> (w443:T6)
    n240 = global read "VAR总磷总氮全局变量.vi" "状态告警区"() -> (w447:T6)
    n241 = Wait (ms)(milliseconds to wait=u32 1000 ("等待时间（毫秒）")) -> ()  [unwired: 1 out]
    n242 = Unbundle By Name(w447) -> ("id"=w421:u16, "flowid"=w420:u16, "量程"=w419:u16, "工作状态"=w423:u16, "日志代码"=w418:u16, "F0"=→"F0":sgl, "F1"=→"F1":sgl, "F2"=→"F2":sgl, "F3"=→"F3":sgl, "ADC"=→"ADC":sgl, "总磷控温温度1"=→"消解温度":sgl, "营养盐控温温度2"=→"注射器温度":sgl)
    n243 = Unbundle By Name(w443) -> ("日志代码"=w442:u16)
    n244 = Unbundle By Name(w446) -> ("日志代码"=w439:u16)
    n245 = Unbundle By Name(w445) -> ("工作状态"=w434:u16, "id"=w435:u16)
    n246 = case shown="0" w434 {
      frame 0 {
        n247 = local write "数组"(string[] [] ("数组")) -> ()
      }
      frame 1, Default {
      }
    }
    n248 = feedback-in #2(w439) -> ()
    n249 = feedback #2(w439) -> (w449:u16)
    n250 = feedback #3(w442) -> (w444:u16)
    n251 = feedback-in #3(w442) -> ()
    n252 = Not Equal To 0?(x=w434) -> (x != 0?=w432:bool)
    n253 = Subtract(x=w439, y=1) -> (x-y=→"多列列表框":i32)
    n254 = Not Equal?(x=w439, y=w449) -> (x != y?=w448:bool)
    n255 = Not Equal?(x=w442, y=w444) -> (x != y?=w441:bool)
    n256 = call <vilib>:"Boolean Crossing PtByPt.vi"("direction"=enum16{"either", "false-true", "true-false"}."false-true", "input"=w432) -> ("crossing"=w436:bool)  [unwired: 1 in]
    n257 = call <vilib>:"Boolean Crossing PtByPt.vi"("direction"=enum16{"either", "false-true", "true-false"}."true-false", "input"=w432) -> ("crossing"=w431:bool)  [unwired: 1 in]
    n258 = Bundle("id"=w421, "flowid"=w420, "量程"=w419) -> (w422:cluster{"id":u16, "flowid":u16, "量程":u16})  [unwired: 1 in]
    n259 = case shown="真" w448 {
      tunnel: w439 -> [_ w618]
      frame False {
      }
      frame True {
        n260 = Subtract(x=w618, y=1) -> (x-y=w616:i32)
        n261 = Subtract(x=w616, y=5) -> (x-y=w620:i32)
        n262 = Greater Or Equal To 0?(x=w620) -> (x >= 0?=w619:bool)
        n263 = property on="多列列表框" class="MCListbox (严格)"() -> (error out=w624:errorcluster, "TopLeft"=w625:T16)  [unwired: 2 in, 1 out]
        n264 = Select(t=w620, s=w619, f=0) -> (s? t:f=w621:i32)
        n265 = Bundle By Name(cluster=w625, "Row"=w621) -> (w626:T16)
        n266 = property on="多列列表框" class="MCListbox (严格)"(error in=w624, "TopLeft"=w626) -> ()  [unwired: 1 in, 2 out]
      }
    }
    n267 = case shown="真" w436 {
      tunnel: w434 -> [_ w489]
      tunnel: w435 -> [_ w486]
      frame False {
      }
      frame True {
        n268 = case shown="8" w489 {
          selector: w489 -> [w496 _ _ _ _ _ _ _ _ _ _ _]
          tunnel: [w495 "【水样测试】" ("字符串") "【标样核查】" ("字符串") "【零点核查】" ("字符串") "【跨度核查】" ("字符串") "【空白测试】" ("字符串") "【平行样测试】" ("字符串") "【加标回收】" ("字符串") "【空白校准】" ("字符串") "【标样校准】" ("字符串") "【单步调试】" ("字符串") "【简易步骤】" ("字符串")] -> w494
          frame 0, Default {
            n269 = Number To Decimal String(number=w496) -> (decimal integer string=w495:string)  [unwired: 1 in]
          }
          frame 1 {
          }
          frame 2 {
          }
          frame 3 {
          }
          frame 4 {
          }
          frame 5 {
          }
          frame 6 {
          }
          frame 7 {
          }
          frame 8 {
          }
          frame 9 {
          }
          frame 254 {
          }
          frame 255 {
          }
        }
        n270 = Concatenate Strings("<<" ("字符串"), w494, "启动" ("字符串")) -> (w493:string)
        n271 = call "id参数转换.vi"("id"=w486) -> ("table输出"=w485:string)  [unwired: 9 in, 1 out]
        n272 = Get Date/Time In Seconds() -> (seconds since 1Jan1904=w491:timestamp)
        n273 = Bundle By Name(cluster=T15 {"时间标识"=timestamp(0 s since 1904-01-01), "设备"="", "日志信息"="", "流程参数"=""} ("data in"), "时间标识"=w491, "设备"=w485, "日志信息"=w493) -> (w490:T15)
        n274 = call "总磷总氮操作日志.vi"("data in"=w490) -> ()  [unwired: 11 in]
      }
    }
    n275 = case shown="真" w431 {
      tunnel: w434 -> [_ w453]
      tunnel: w435 -> [_ w466]
      frame False {
      }
      frame True {
        n276 = case shown="6" w453 {
          selector: w453 -> [w473 _ _ _ _ _ _ _ _ _ _ _]
          tunnel: [w472 "【水样测试】" ("字符串") "【标样核查】" ("字符串") "【零点核查】" ("字符串") "【跨度核查】" ("字符串") "【空白测试】" ("字符串") "【平行样测试】" ("字符串") "【加标回收】" ("字符串") "【空白校准】" ("字符串") "【标样校准】" ("字符串") "【单步调试】" ("字符串") "【简易步骤】" ("字符串")] -> w454
          frame 0, Default {
            n277 = Number To Decimal String(number=w473) -> (decimal integer string=w472:string)  [unwired: 1 in]
          }
          frame 1 {
          }
          frame 2 {
          }
          frame 3 {
          }
          frame 4 {
          }
          frame 5 {
          }
          frame 6 {
          }
          frame 7 {
          }
          frame 8 {
          }
          frame 9 {
          }
          frame 254 {
          }
          frame 255 {
          }
        }
        n278 = global read "VAR总磷总氮全局变量.vi" "状态告警区"() -> (w464:T6)
        n279 = Unbundle By Name(w464) -> ("F0"=w463:sgl, "F1"=w462:sgl, "F2"=w461:sgl, "F3"=w460:sgl, "id"=w459:u16, "flowid"=w458:u16, "量程"=w457:u16)
        n280 = Concatenate Strings(w454, "停止" ("字符串"), ">>" ("字符串")) -> (w471:string)
        n281 = Format Into String(format string="F0=%#f,F1=%#f,F2=%#f,F3=%#f,Flow=%d-%-d-%-d" ("格式字符串"), w463, w462, w461, w460, w459, w458, w457) -> (resulting string=w455:string)  [unwired: 2 in, 1 out]
        n282 = call "id参数转换.vi"("id"=w466) -> ("table输出"=w465:string)  [unwired: 9 in, 1 out]
        n283 = Get Date/Time In Seconds() -> (seconds since 1Jan1904=w469:timestamp)
        n284 = Bundle By Name(cluster=T15 {"时间标识"=timestamp(0 s since 1904-01-01), "设备"="", "日志信息"="", "流程参数"=""} ("data in"), "时间标识"=w469, "设备"=w465, "日志信息"=w471, "流程参数"=w455) -> (w468:T15)
        n285 = call "总磷总氮操作日志.vi"("data in"=w468) -> ()  [unwired: 11 in]
      }
    }
    n286 = case shown="真" w441 {
      frame False {
      }
      frame True {
        n287 = property on="多列列表框" class="MCListbox (严格)"() -> ("ItemNames"=w513:string[][], "Value"=w509:i32)  [unwired: 2 in, 2 out]
        n288 = Index Array(array=w513, index (row)=w509) -> (element=w512:string[])  [unwired: 1 in]
        n289 = Index Array(array=w512) -> (element=w511:string)  [unwired: 1 in]
        n290 = call "过滤筛选流程.vi"("字符串"=w511) -> ("匹配后偏移量"=w510:i32)  [unwired: 10 in]
        n291 = case shown="默认" w510 {
          tunnel: w511 -> [w515 _]
          tunnel: w509 -> [w514 _]
          frame Default {
            n292 = case shown="默认" w515 {
              selector: w515 -> [w521 w528]
              tunnel: [w521 w528] -> w517
              tunnel: [string[] [] ("数组") w523] -> w516
              tunnel: w514 -> [_ w527]
              frame "读数" {
              }
              frame Default {
                n293 = Equal?(x=w527, y=1) -> (x = y?=w525:bool)
                n294 = Select(t=string[] [], s=w525, f="数组") -> (s? t:f=w523:string[])
              }
            }
            n295 = for {
              N: 1 -> [_]
              tunnel: w517 -> [w530]
              shift-right: [w529] -> w518
              shift-left: w516 -> [w531]
              n296 = Search 1D Array(1D array=w531, element=w530) -> (index of element=w534:i32)  [unwired: 1 in]
              n297 = Format Into String(format string="%s" ("格式字符串"), w530) -> (resulting string=w535:string)  [unwired: 2 in, 1 out]
              n298 = Equal?(x=w534, y=-1) -> (x = y?=w532:bool)
              n299 = case shown="真" w532 {
                tunnel: w535 -> [_ w545]
                tunnel: w531 -> [w537 w549]
                tunnel: w530 -> [_ w548]
                tunnel: [w537 w547] -> w529
                frame False {
                }
                frame True {
                  n300 = case shown="\"结束\"" w545 {
                    selector: w545 -> [w579 w582 w585]
                    tunnel: [w579 w581 w584] -> w544
                    frame Default {
                    }
                    frame "初始化" {
                      n301 = Concatenate Strings("<<--" ("字符串"), w582) -> (w581:string)
                    }
                    frame "结束" {
                      n302 = Concatenate Strings("-->>" ("字符串"), w585) -> (w584:string)
                    }
                  }
                  n303 = Insert Into Array(array=w549, new element=w548) -> (w547:string[])  [unwired: 1 in]
                  n304 = global read "VAR总磷总氮全局变量.vi" "状态告警区"() -> (w543:T6)
                  n305 = Unbundle By Name(w543) -> ("工作状态"=w542:u16)
                  n306 = case shown="0, 默认" w542 {
                    selector: w542 -> [w564 _ _ _ _ _ _ _ _ _ _ _]
                    tunnel: [w563 "【水样测试】" ("字符串") "【标样核查】" ("字符串") "【零点核查】" ("字符串") "【跨度核查】" ("字符串") "【空白测试】" ("字符串") "【平行样测试】" ("字符串") "【加标回收】" ("字符串") "【空白校准】" ("字符串") "【标样校准】" ("字符串") "【单步调试】" ("字符串") w575] -> w540
                    frame 0, Default {
                      n307 = Number To Decimal String(number=w564) -> (decimal integer string=w563:string)  [unwired: 1 in]
                    }
                    frame 1 {
                    }
                    frame 2 {
                    }
                    frame 3 {
                    }
                    frame 4 {
                    }
                    frame 5 {
                    }
                    frame 6 {
                    }
                    frame 7 {
                    }
                    frame 8 {
                    }
                    frame 9 {
                    }
                    frame 254 {
                    }
                    frame 255 {
                      n308 = local read "简易步骤名称"() -> (w577:string)
                      n309 = Format Into String(format string="(%s)" ("格式字符串"), initial string="【简易流程】" ("工作状态"), w577) -> (resulting string=w575:string)  [unwired: 1 in, 1 out]
                    }
                  }
                  n310 = global read "VAR总磷总氮全局变量.vi" "状态告警区"() -> (w562:T6)
                  n311 = global read "VAR总磷总氮全局变量.vi" "状态告警区"() -> (w559:T6)
                  n312 = Unbundle By Name(w559) -> ("F0"=w556:sgl, "F1"=w555:sgl, "F2"=w554:sgl, "F3"=w553:sgl, "id"=w552:u16, "flowid"=w551:u16, "量程"=w550:u16)
                  n313 = Unbundle By Name(w562) -> ("id"=w539:u16)
                  n314 = call "id参数转换.vi"("id"=w539) -> ("table输出"=w538:string)  [unwired: 9 in, 1 out]
                  n315 = Concatenate Strings(w540, w544) -> (w541:string)
                  n316 = Format Into String(format string="F0=%#f,F1=%#f,F2=%#f,F3=%#f,Flow=%d-%-d-%-d" ("格式字符串"), w556, w555, w554, w553, w552, w551, w550) -> (resulting string=w557:string)  [unwired: 2 in, 1 out]
                  n317 = Get Date/Time In Seconds() -> (seconds since 1Jan1904=w560:timestamp)
                  n318 = Bundle By Name(cluster=T15 {"时间标识"=timestamp(0 s since 1904-01-01), "设备"="", "日志信息"="", "流程参数"=""} ("data in"), "时间标识"=w560, "设备"=w538, "日志信息"=w541, "流程参数"=w557) -> (w561:T15)
                  n319 = call "总磷总氮操作日志.vi"("data in"=w561) -> ()  [unwired: 11 in]
                }
              }
            }
            n320 = local write "数组"(w518) -> ()
          }
          frame -1 {
          }
        }
      }
    }
    n321 = while {
      tunnel: w422 -> [w600]
      shift-right: [w595] -> _
      shift-left: _ -> [w597]
      shift-right: [w596] -> _
      shift-left: _ -> [w598]
      shift-right: [w587] -> _
      shift-left: _ -> [w594]
      tunnel: w423 -> [w586]
      shift-right: [w592] -> _
      shift-left: _ -> [w591]
      tunnel: w418 -> [w592]
      stop <- TRUE stop-if-true
      n322 = case shown="255" w586 {
        tunnel: [w601 w602] -> w587
        frame 0, Default {
          n323 = global read "总磷总氮断电保存全局变量.vi" "流程路径"() -> (w601:path)
        }
        frame 255 {
          n324 = global read "总磷总氮断电保存全局变量.vi" "简易流程路径"() -> (w602:path)
        }
      }
      n325 = Not Equal?(x=w591, y=w592) -> (x != y?=w590:bool)
      n326 = Not Equal To 0?(x=w586) -> (x != 0?=w588:bool)
      n327 = Not Equal?(x=w594, y=w587) -> (x != y?=w589:bool)
      n328 = Compound Arithmetic op=OR ("复合运算")(w588, w589, w590) -> (w593:bool)
      n329 = case shown="真" w593 {
        tunnel: [w604 w614] -> w596
        tunnel: [w603 w613] -> w595
        tunnel: w600 -> [_ w608]
        tunnel: w598 -> [w604 _]
        tunnel: w597 -> [w603 _]
        tunnel: w587 -> [_ w607]
        tunnel: w586 -> [_ w606]
        frame False {
        }
        frame True {
          n330 = call "斯坦道XML解析.vi"("工作状态"=w606, "添加的路径"=w607, "参数簇"=w608) -> ("简易步骤名称"=→"简易步骤名称":string, "步骤时间"=w609:string[], "步骤名"=w611:string[])  [unwired: 6 in]
          n331 = for {
            tunnel: w611 -> [_] mode=indexing
            tunnel: [w615] -> w612 mode=indexing
            i -> [w615]
          }
          n332 = Build Array(w611, w609) -> (w610:string[][])
          n333 = Transpose 2D Array(2D array=w610) -> (transposed array=w613:string[][])
          n334 = Number To Decimal String(number=w612) -> (decimal integer string=w614:string[])  [unwired: 1 in]
        }
      }
      n335 = property on="多列列表框" class="MCListbox (严格)"("ItemNames"=w595, "RowHdrs[]"=w596) -> ()  [unwired: 2 in, 2 out]
    }
  }
  n336 = Search/Split String(string=w18, search string/char (-)="." ("搜索字符串/字符(-)")) -> (substring before match=w16:string)  [unwired: 1 in, 2 out]
  n337 = call <vilib>:"Application Directory.vi"() -> ("Application Directory"=w22:path)
  n338 = Concatenate Strings(w16, "-" ("字符串"), "calibration.xml" ("名称或相对路径")) -> (w13:string)
  n339 = Build Path(base path=w22, name or relative path="data" ("名称或相对路径")) -> (appended path=w19:path)
  n340 = Build Path(base path=w19, name or relative path=w13) -> (appended path=w12:path)
  n341 = while {
    shift-right: [w630] -> _
    shift-left: _ -> [w632]
    tunnel: w12 -> [w629]
    tunnel: [w627] -> _
    stop <- FALSE stop-if-true
    n342 = Read from Text File(file (use dialog)=w629) -> (text=w630:string, error out=w627:errorcluster)  [unwired: 3 in, 2 out]
    n343 = Wait (ms)(milliseconds to wait=u32 1000 ("等待时间（毫秒）")) -> ()  [unwired: 1 out]
    n344 = Not Equal?(x=w632, y=w630) -> (x != y?=w631:bool)
    n345 = case shown="真" w631 {
      tunnel: w629 -> [_ _]
      tunnel: [_ w634] -> _
      frame False {
      }
      frame True {
        n346 = call "读取校准数据.vi"() -> ("错误输出"=w634:errorcluster)  [unwired: 11 in]
      }
    }
  }
  n347 = while {
    shift-right: [w638] -> _
    shift-left: 0 -> [w639]
    stop <- FALSE stop-if-true
    n348 = local read "关闭心跳包"() -> (w640:bool)
    n349 = Wait (ms)(milliseconds to wait=u32 1000 ("等待时间（毫秒）")) -> ()  [unwired: 1 out]
    n350 = case shown="真" w640 {
      tunnel: w639 -> [_ w644]
      tunnel: [_ w643] -> w638
      frame False {
      }
      frame True {
        n351 = Increment(x=w644) -> (x+1=w643:i32)
      }
    }
    n352 = Greater Or Equal?(x=w638, y=300) -> (x >= y?=w636:bool)
    n353 = case shown="真" w636 {
      frame False {
      }
      frame True {
        n354 = local write "关闭心跳包"(FALSE ("关闭心跳包")) -> ()
      }
    }
  }
  n355 = vi-ref "校准设置页.vi"() -> (w7:refnum<vi>)
  n356 = vi-ref "参数设置页.vi"() -> (w11:refnum<vi>)
  n357 = property class="VI"(reference=w7, error in=w2) -> (reference out=w5:refnum<vi>, "Exec.State"=w6:T7)  [unwired: 1 out]
  n358 = property class="VI"(reference=w11, error in=w3) -> (reference out=w9:refnum<vi>, "Exec.State"=w10:T7)  [unwired: 1 out]
  n359 = case shown="\"Bad\", 默认" w6 {
    tunnel: w5 -> [w645 w649]
    tunnel: [w645 w646] -> w4
    frame "Bad", Default {
    }
    frame "Idle" {
      n360 = invoke class="VI" method="Run VI"(reference=w649, "Wait until done"=FALSE ("结束前等待"), "Auto Dispose Ref"=TRUE ("自动销毁引用")) -> (reference out=w646:refnum<vi>)  [unwired: 2 in, 4 out]
    }
  }
  n361 = case shown="\"Bad\", 默认" w10 {
    tunnel: w9 -> [w650 w654]
    tunnel: [w650 w651] -> w8
    frame "Bad", Default {
    }
    frame "Idle" {
      n362 = invoke class="VI" method="Run VI"(reference=w654, "Wait until done"=FALSE ("结束前等待"), "Auto Dispose Ref"=TRUE ("自动销毁引用")) -> (reference out=w651:refnum<vi>)  [unwired: 2 in, 4 out]
    }
  }
  n363 = Obtain Notifier(name (unnamed)=w28, notification data type=FALSE) -> (notifier out=w29:refnum<notifier>)  [unwired: 2 in, 2 out]
  n364 = Obtain Queue(name (unnamed)=w28, element data type=cluster{"命令":string, "data":variant} {"命令"="", "data"=variant}) -> (queue out=w33:refnum<queue>)  [unwired: 3 in, 2 out]
  n365 = while {
    tunnel: w33 -> [w658]
    tunnel: w29 -> [w657]
    tunnel: w8 -> [w656]
    tunnel: w4 -> [w655]
    stop <- FALSE stop-if-true
    n366 = event shown="[8] \"调试\": 值改变" {
      selector: _ -> [_ _ _ _ _ _ _ _ _ _ _ _ _]
      dyn-events: _ -> [_ _ _ _ _ _ _ _ _ _ _ _ _]
      timeout: _ -> [_ _ _ _ _ _ _ _ _ _ _ _ _]
      tunnel: w658 -> [_ _ _ _ _ _ _ w666 _ w675 _ _ _]
      tunnel: w657 -> [_ _ _ _ _ _ _ _ _ w671 _ _ _]
      tunnel: w656 -> [_ _ _ _ _ _ _ _ _ _ w676 _ _]
      tunnel: w655 -> [_ _ _ _ _ _ _ _ _ _ _ w679 _]
      event Timeout {
        n367 = event-data() -> ()  [unwired: 1 in, 3 out]
      }
      event "温度曲线": Value Change {
        n368 = event-data() -> ()  [unwired: 1 in, 6 out]
        n369 = call "温度曲线显示.vi"() -> ()  [unwired: 12 in]
      }
      event "试剂余量": Value Change {
        n370 = event-data() -> ()  [unwired: 1 in, 6 out]
        n371 = call "试剂余量显示UI.vi"() -> ()  [unwired: 12 in]
      }
      event "灯值调整": Value Change {
        n372 = event-data() -> ()  [unwired: 1 in, 6 out]
        n373 = call "灯值调整对话框.vi"() -> ()  [unwired: 12 in]
      }
      event "启动参数设置": Value Change {
        n374 = event-data() -> ()  [unwired: 1 in, 6 out]
        n375 = call "启动参数设置.vi"() -> ()  [unwired: 12 in]
      }
      event "布尔": Mouse Down {
        n376 = event-data() -> ("CtlRef"=w661:refnum<vi>)  [unwired: 1 in, 5 out]
        n377 = property class="Bool (严格)"(reference=w661) -> ("Value"=w660:bool)  [unwired: 1 in, 2 out]
        n378 = case shown="假" w660 {
          frame False {
            n379 = call "密码键盘.vi"() -> ("NewNumber"=w662:u32)  [unwired: 1 in]
            n380 = global write "VAR总磷总氮全局变量.vi" "权限密码"(w662) -> ()
          }
          frame True {
            n381 = global write "VAR总磷总氮全局变量.vi" "权限密码"(u32 0 ("输入密码")) -> ()
          }
        }
      }
      event "流程固件": Value Change {
        n382 = event-data() -> ()  [unwired: 1 in, 6 out]
        n383 = call "流程固件设置对话框.vi"() -> ()  [unwired: 12 in]
      }
      event "手动启动": Value Change {
        n384 = event-data() -> ()  [unwired: 1 in, 6 out]
        n385 = call "总磷总氮启动参数对话框.vi"() -> ("确认"=w664:bool, "元素"=w665:cluster{"命令":string, "data":variant})  [unwired: 10 in]
        n386 = case shown="真" w664 {
          tunnel: w666 -> [_ w669]
          tunnel: w665 -> [_ w668]
          frame False {
          }
          frame True {
            n387 = Flush Queue(queue=w669) -> (queue out=w667:refnum<queue>)  [unwired: 1 in, 2 out]
            n388 = Enqueue Element(queue=w667, element=w668) -> ()  [unwired: 2 in, 3 out]
          }
        }
      }
      event "调试": Value Change {
        n389 = event-data() -> ()  [unwired: 1 in, 6 out]
        n390 = call "简易流程调试界面.vi"() -> ()  [unwired: 12 in]
      }
      event "停止": Value Change {
        n391 = event-data() -> ()  [unwired: 1 in, 6 out]
        n392 = Send Notification(notification=TRUE ("通知"), notifier=w671) -> ()  [unwired: 1 in, 2 out]
        n393 = Enqueue Element(queue=w675, element=cluster{"命令":string, "data":variant} {"命令"="启动", "data"=variant(cluster{"站号":u16, "控制命令输出":u16[]} {"站号"=1, "控制命令输出"=[2816]})} ("元素")) -> (queue out=w672:refnum<queue>)  [unwired: 2 in, 2 out]
        n394 = Enqueue Element(queue=w672, element=cluster{"命令":string, "data":variant} {"命令"="启动", "data"=variant(cluster{"站号":u16, "控制命令输出":u16[]} {"站号"=2, "控制命令输出"=[2816]})} ("元素")) -> ()  [unwired: 2 in, 3 out]
      }
      event "参数设置", "参数查询": Value Change {
        n395 = event-data() -> ()  [unwired: 1 in, 6 out]
        n396 = property on="窗格" class="Pane"("Origin"=T8 {"Horizontal"=0, "Vertical"=640} ("原点")) -> ()  [unwired: 2 in, 2 out]
        n397 = invoke on="子面板" class="SubPnl" method="Remove VI"() -> (error out=w677:errorcluster)  [unwired: 3 in, 2 out]
        n398 = invoke on="子面板" class="SubPnl" method="Insert VI"(error in=w677, "VI Ref"=w676) -> ()  [unwired: 2 in, 4 out]
      }
      event "仪器校准": Value Change {
        n399 = event-data() -> ()  [unwired: 1 in, 6 out]
        n400 = invoke on="子面板" class="SubPnl" method="Remove VI"() -> (error out=w680:errorcluster)  [unwired: 3 in, 2 out]
        n401 = invoke on="子面板" class="SubPnl" method="Insert VI"(error in=w680, "VI Ref"=w679) -> ()  [unwired: 2 in, 4 out]
      }
      event "返回": Value Change {
        n402 = event-data() -> ()  [unwired: 1 in, 6 out]
        n403 = property on="窗格" class="Pane"("Origin"=T8 {"Horizontal"=0, "Vertical"=0} ("原点")) -> ()  [unwired: 2 in, 2 out]
      }
    }
  }
  n404 = while {
    tunnel: w33 -> [w692]
    stop <- FALSE stop-if-true
    n405 = Wait (ms)(milliseconds to wait=u32 1000 ("等待时间（毫秒）")) -> ()  [unwired: 1 out]
    n406 = global read "总磷总氮断电保存全局变量.vi" "MB通信方式选择"() -> (w690:enum16{"串口", "TCP"})
    n407 = global read "VAR总磷总氮全局变量.vi" "MB session in"() -> (w688:refnum<class "MB_Master.lvclass">)
    n408 = Get Queue Status(queue=w692) -> (queue out=w691:refnum<queue>, # elements in queue=w687:i32)  [unwired: 2 in, 6 out]
    n409 = case shown="\"串口\", 默认" w690 {
      tunnel: [w695 w696] -> w689
      frame "串口", Default {
        n410 = global read "总磷总氮断电保存全局变量.vi" "VISA Resource"() -> (w695:refnum<visa-resource-name>)
      }
      frame "TCP" {
        n411 = global read "总磷总氮断电保存全局变量.vi" "IP"() -> (w696:string)
      }
    }
    "字符串 2" <- w689
    n412 = property class="MB_Master"(reference=w688) -> ("Properties:Session Valid"=w686:bool)  [unwired: 1 in, 2 out]
    n413 = Equal To 0?(x=w687) -> (x = 0?=w685:bool)
    n414 = Not(x="关闭心跳包") -> (.not. x?=w683:bool)
    n415 = Compound Arithmetic op=AND ("复合运算")(w685, w686, w683) -> (w682:bool)
    n416 = global write "VAR总磷总氮全局变量.vi" "心跳包打开状态"(w682) -> ()
    n417 = case shown="真" w682 {
      tunnel: w691 -> [_ w708]
      frame False {
      }
      frame True {
        n418 = global read "总磷总氮断电保存全局变量.vi" "启动队列名称"() -> (w697:cluster{"String":string, "Value":u16}[])
        n419 = for {
          tunnel: [w726] -> w698 mode=indexing
          tunnel: w697 -> [w727] mode=indexing
          n420 = Unbundle By Name(w727) -> ("Value"=w726:u16)
        }
        n421 = global read "VAR总磷总氮全局变量.vi" "状态告警区"() -> (w700:T6)
        n422 = Unbundle By Name(w700) -> ("系统时间"=w707:timestamp, "工作状态"=w699:u16)
        n423 = Get Date/Time In Seconds() -> (seconds since 1Jan1904=w706:timestamp)
        n424 = for {
          tunnel: w699 -> [w712]
          shift-right: [w713] -> w701
          shift-left: w708 -> [w715]
          tunnel: w698 -> [w709] mode=indexing
          n425 = Equal?(x=w712, y=T17."空闲") -> (x = y?=w710:bool)
          n426 = Bundle By Name(cluster=cluster{"命令":string, "data":variant} {"命令"="", "data"=variant} ("元素"), "命令"="读状态告警区", "data"=w709) -> (w717:cluster{"命令":string, "data":variant})
          n427 = Enqueue Element(queue=w715, element=w717) -> (queue out=w714:refnum<queue>)  [unwired: 2 in, 2 out]
          n428 = case shown="真" w710 {
            tunnel: w714 -> [w719 w722]
            tunnel: w709 -> [_ w721]
            tunnel: [w719 w720] -> w713
            frame False {
            }
            frame True {
              n429 = Bundle By Name(cluster=cluster{"命令":string, "data":variant} {"命令"="", "data"=variant} ("元素"), "命令"="读测量数据区", "data"=w721) -> (w724:cluster{"命令":string, "data":variant})
              n430 = Enqueue Element(queue=w722, element=w724) -> (queue out=w720:refnum<queue>)  [unwired: 2 in, 2 out]
            }
          }
        }
        n431 = Subtract(x=w706, y=w707) -> (x-y=w705:dbl)
        n432 = Absolute Value(x=w705) -> (abs(x)=w704:dbl)
        n433 = Greater Or Equal?(x=w704, y=120.0) -> (x >= y?=w702:bool)
        n434 = case shown="真" w702 {
          tunnel: w701 -> [_ w735]
          tunnel: [w728 _] -> _
          frame False {
            n435 = global read "VAR总磷总氮全局变量.vi" "MB session in"() -> (w733:refnum<class "MB_Master.lvclass">)
            n436 = call "序列号读取.vi"("MB session in"=w733) -> ("error out"=w731:errorcluster, "序列号"=w732:string, "MB session out"=w730:refnum<class "MB_Master.lvclass">)  [unwired: 8 in]
            n437 = global write "VAR总磷总氮全局变量.vi" "序列号"(w732) -> ()
            n438 = call "总磷总氮版本号读取.vi"("Error in"=w731, "MB session in"=w730) -> ("error out"=w728:errorcluster, "固件版本号"=→"固件版本号":string)  [unwired: 7 in, 1 out]
          }
          frame True {
            n439 = call "总磷总氮启动命令.vi"("参数"=T18 {"站号"=3, "量程切换"=enum."AUTO", "控制命令"=enum."校时", "模式设置"=enum."待机", "测量间隔"=0}) -> ("启动命令"=w734:cluster{"命令":string, "data":variant})  [unwired: 10 in]
            n440 = Enqueue Element(queue=w735, element=w734) -> ()  [unwired: 2 in, 3 out]
          }
        }
      }
    }
  }
